vi "PID Motor C0.vi"(6 "PID gains":T2={"proportional gain (Kc)"=0.05, "integral time (Ti, min)"=0.003, "derivative time (Td, min)"=0.0} {"derivative time (Td, min)" format="%.6f"; "integral time (Ti, min)" format="%.6f"; "proportional gain (Kc)" format="%.6f"}, 7 "reinitialize? (F)":bool, 8 "error in (no error)":errorcluster, 9 "input":dbl, 10 "dt in (ms)":i32=-1, 11 "Setpoint C0":dbl(slide)=-0.016713091922005565 scale=-2.0..2.0) -> (0 "error out":errorcluster, 1 "dx/dt":dbl, 2 "output":dbl format="%.2f", 3 "Speed C0":T1(graph), 4 "dt out (s)":dbl format="%.3f", 5 "Counter C0":dbl)   [LabVIEW 2017]
uses:
  <vilib>/myRIO/Instrument Drivers/Onboard IO/PWM/typedefs/PWM Reference.ctl
  <vilib>/myRIO/Common/Instrument Driver Framework/Utilities/typedefs/myRIO Generic Hardware Reference.ctl
  <vilib>/myRIO/Common/Instrument Driver Framework/Utilities/typedefs/Hardware Version Enum.ctl
  <vilib>/myRIO/Common/Instrument Driver Framework/Utilities/typedefs/myRIO v1.0 Reference.ctl
  <vilib>/myRIO/Common/Instrument Driver Framework/Utilities/typedefs/Generic FPGA Reference.ctl
  <vilib>/myRIO/Common/Instrument Driver Framework/myRIO v1.0/PWM/typedefs/PWM Channels Enum.ctl
  <vilib>/myRIO/Instrument Drivers/Onboard IO/PWM/typedefs/PWM Configuration.ctl
  <vilib>/userdefined/High Color/nirio_resource_hc.ctl
  <vilib>/myRIO/Common/Instrument Driver Framework/Utilities/vis/Is FPGA Ref Available.vi
  <vilib>/myRIO/Common/Instrument Driver Framework/myRIO v1.0/PWM/vis/myRIO v1.1 Open PWM.vi
  <vilib>/myRIO/Instrument Drivers/Onboard IO/PWM/vis/Set Duty Cycle and Frequency.vi
  <vilib>/myRIO/Common/Instrument Driver Framework/Utilities/vis/Validate Channels.vi
  <vilib>/myRIO/Common/Instrument Driver Framework/myRIO v1.0/PWM/vis/myRIO v1.0 Reserve PWM.vi
  <vilib>/myRIO/Common/Instrument Driver Framework/myRIO v1.0/PWM/vis/myRIO v1.0 Build MUX Configuration PWM.vi
  <vilib>/myRIO/Common/Instrument Driver Framework/myRIO v1.0/Resource Manager/vis/myRIO v1.0 Reserve Channel List.vi
  <vilib>/myRIO/Common/Instrument Driver Framework/myRIO v1.0/Resource Manager/vis/myRIO v1.0 Create Configuration List.vi
  <vilib>/myRIO/Common/Instrument Driver Framework/myRIO v1.0/Resource Manager/vis/myRIO v1.0 Reserve Channel.vi
  <vilib>/myRIO/Common/Instrument Driver Framework/myRIO v1.0/Resource Manager/vis/myRIO v1.0 Unreserve Channel.vi
  <vilib>/myRIO/Common/Instrument Driver Framework/myRIO v1.0/Resource Manager/vis/myRIO v1.0 Build Mutex Name.vi
  <vilib>/Utility/VariantDataType/GetNumericInfo.vi
  <vilib>/Utility/error.llb/Error Cluster From Error Code.vi
  <vilib>/myRIO/Common/Instrument Driver Framework/myRIO v1.0/myRIO v1.1 Open.vi
  <vilib>/myRIO/Common/Instrument Driver Framework/Utilities/vis/IO Manager.vi
  <vilib>/myRIO/Common/Instrument Driver Framework/Utilities/vis/Configuration Manager.vi
  <vilib>/myRIO/Common/Instrument Driver Framework/myRIO v1.0/Resource Manager/vis/myRIO v1.0 Configure IO.vi
  <vilib>/myRIO/Common/Instrument Driver Framework/myRIO v1.0/myRIO v1.0 Close.vi
  <vilib>/myRIO/Common/Instrument Driver Framework/myRIO v1.0/PWM/vis/myRIO v1.0 Write PWM.vi
  <vilib>/addons/control/pid/pid.llb/PID (DBL).vi
  <vilib>/myRIO/Express VI/Onboard IO/PWM/PWM Express VI.xnode
  <vilib>/myRIO/Instrument Drivers/Onboard IO/PWM/vis/myRIO PWM Open.xnode
  <vilib>/addons/control/pid/NI_PID_pid.lvlib
  <vilib>/myRIO/Instrument Drivers/Onboard IO/PWM/PWM.lvlib
panel:
  in  "Encoder accuracy multiplier":dbl=1.0
  # "VI Description: Converts the input into a PWM value to move the motor, measures the velocity of a motor,\nthen recalculates the new input (in the form of the output)"
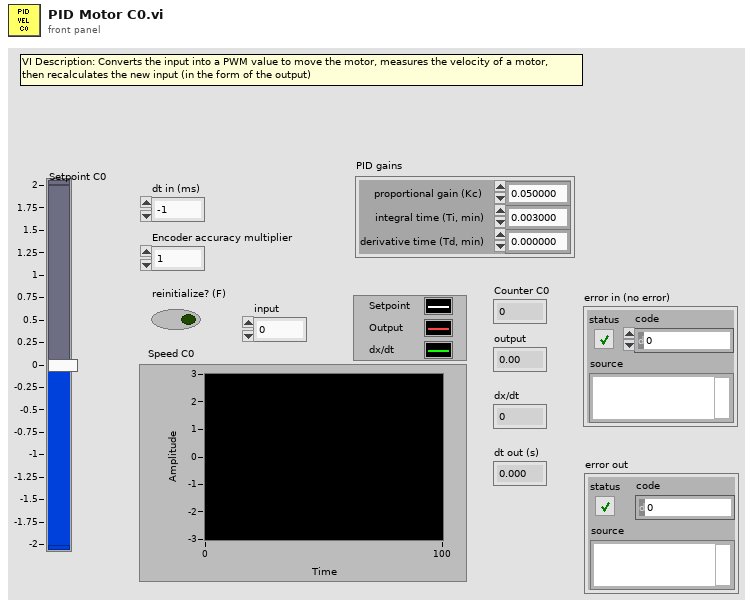
[diagram p1: front panel]
types:
  T1 = cluster{"Setpoint":dbl, "output":dbl, "dx/dt":dbl}
  T2 = cluster{"proportional gain (Kc)":dbl, "integral time (Ti, min)":dbl, "derivative time (Td, min)":dbl}
  T3 = cluster{"Setpoint C0":dbl, "output":dbl, "dx/dt":dbl}
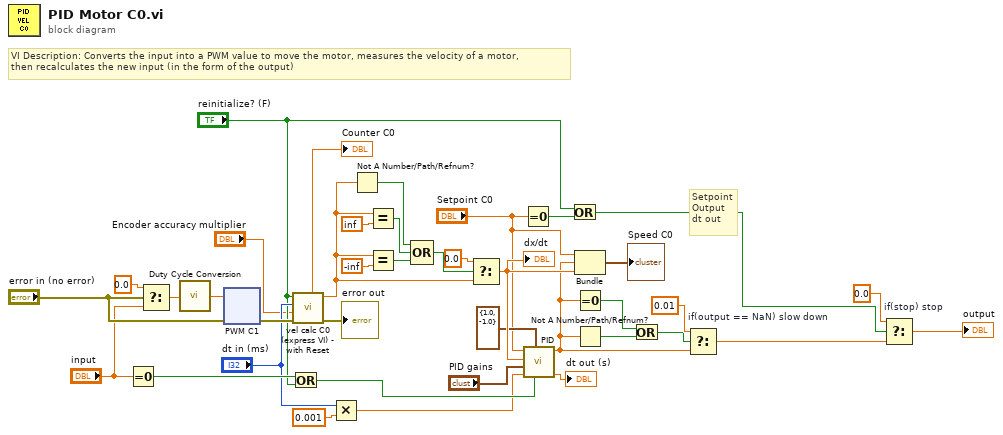
[diagram p0: block diagram]
diagram:
  # "VI Description: Converts the input into a PWM value to move the motor, measures the velocity of a motor,\nthen recalculates the new input (in the form of the output)"
  # "Setpoint\nOutput\ndt out"
  n1 = Equal To 0?(x="input") -> (x = 0?=w28:bool)
  n2 = Select(t=0.0, s="error in (no error)", f="input") -> (s? t:f=w2:dbl)
  n3 = call "Duty Cycle Conversion.vi"("Duty Cycle In"=w2) -> ("Duty Cyle Out"=w32:dbl)
  n4 = xnode "PWM C1"("error in (no error)"="error in (no error)", "Duty Cycle"=w32) -> ("error out"=w31:errorcluster)
  n5 = Or(x=w28, y="reinitialize? (F)") -> (x .or. y?=w27:bool)
  n6 = call "vel calc C0 (express VI) - with Reset.vi"("error in"=w31, "Encoder accuracy multiplier"="Encoder accuracy multiplier", "dt in (ms)"="dt in (ms)", "Reinitialise"="reinitialize? (F)") -> ("error out"=→"error out":errorcluster, "dx/dt"=w17:dbl, "Counter Value"=→"Counter C0":dbl)  [unwired: 3 in, 2 out]
  n7 = Multiply(x="dt in (ms)", y=0.001) -> (x*y=w24:dbl)
  n8 = Not A Number/Path/Refnum?(number/path/refnum=w17) -> (NaN/Path/Refnum?=w19:bool)
  n9 = Equal?(x=w17, y=inf) -> (x = y?=w20:bool)
  n10 = Equal?(x=w17, y=-inf) -> (x = y?=w21:bool)
  n11 = Compound Arithmetic op=OR(w19, w20, w21) -> (w18:bool)
  n12 = Select(t=0.0, s=w18, f=w17) -> (s? t:f=w39:dbl)
  "dx/dt" <- w39
  n13 = Equal To 0?(x="Setpoint C0") -> (x = 0?=w11:bool)
  n14 = call-poly <vilib>:"PID.vi"("reinitialize? (F)"=w27, "output range"=cluster{"output high":dbl, "output low":dbl} {"output high"=1.0, "output low"=-1.0}, "dt (s)"=w24, "PID gains"="PID gains", "process variable"=w39, "setpoint"="Setpoint C0") -> ("dt out (s)"=→"dt out (s)":dbl, "output"=w9:dbl)  [unwired: 4 in]
  n15 = Or(x="reinitialize? (F)", y=w11) -> (x .or. y?=w10:bool)
  n16 = Bundle("Setpoint C0"="Setpoint C0", "output"=w9, "dx/dt"=w39) -> (→"Speed C0":T3)  [unwired: 1 in]
  n17 = Equal To 0?(x=w9) -> (x = 0?=w8:bool)
  n18 = Not A Number/Path/Refnum?(number/path/refnum=w9) -> (NaN/Path/Refnum?=w7:bool)
  n19 = Or(x=w8, y=w7) -> (x .or. y?=w6:bool)
  n20 = Select "if(output == NaN) slow down"(t=0.01, s=w6, f=w9) -> (s? t:f=w16:dbl)
  n21 = Select "if(stop) stop"(t=0.0, s=w10, f=w16) -> (s? t:f=→"output":dbl)
